vi "Unibot cRIO.vi"() -> ()   [LabVIEW 2012]
uses:
  Unibot - State Machine Controller.vi
  <vilib>/Simulation/Implementation/XNodeFramework/SimXNode/SimX.xnode
  Unibot - Nonlinear Model.vi
  <vilib>/Simulation/Utility/Implementation/SIM Halt.vi
  <vilib>/Simulation/SignalDisplay/Implementation/NILVSim Time Waveform.llb/SIM Time Waveform (scalar).vi
  <vilib>/Simulation/Implementation/Shared/SIMSCR Execution Mode.ctl
  <vilib>/Simulation/Scripting/Companion Diagram/SimConfigNode/_simSolvers.ctl
  <vilib>/Simulation/Scripting/Companion Diagram/SimConfigNode/SimParams.ctl
  <vilib>/Simulation/Scripting/Companion Diagram/SimConfigNode/SimDog.xnode
panel:
  in  "Tab Control":T1(tab)
  in  "Start Open Loop":bool
  out "torque 2":waveform(dbl)(graph)={"t0"=timestamp(0 s since 1904-01-01), "dt"=1.0, "Y"=[0.0]}
  out "teta2 2":waveform(dbl)(graph)={"t0"=timestamp(0 s since 1904-01-01), "dt"=1.0, "Y"=[0.0]}
  out "teta1 2":waveform(dbl)(graph)={"t0"=timestamp(0 s since 1904-01-01), "dt"=1.0, "Y"=[0.0]}
  in  "Initial Theta1 (Elbow)":dbl(knob) scale=-3.14..3.14
  in  "Initial Theta2 (Arm)":dbl(knob) scale=-3.14..3.14
  in  "Right":bool
  in  "Intensity":dbl(slide)=10.0 scale=0.0..10.0
  in  "Left":bool
  in  "Control Technique":T2(tab)
  in  "Q":dbl[][](array[numeric])=[[10.0, 0.0, 0.0, 0.0], [0.0, 10.0, 0.0, 0.0], [0.0, 0.0, 100.0, 0.0], [0.0, 0.0, 0.0, 1.0]] format="%.2f"
  in  "R":dbl[][](array[numeric])=[[50.0]] format="%.2f"
  in  "Desired Pole Location":cdb[](array[numeric])=[0.8275428216771237+0.0i, 0.9068860314786581+0.0i, 0.9511525717602396+0.0i, 0.9425028249515996+0.0i] format="%.2f"
  out "Optimal Gain \nDown-Up":dbl[](array[numeric])=[13.362365480735772, 19.05380394095224, 1.2104119144158012, 2.4013527998190582] format="%.2f"
  out "Optimal Gain\nDown-Down":dbl[](array[numeric])=[-0.14906178101626644, 0.17686358569380023, 1.1761652926773682, -0.039275718443801] format="%.2f"
  out "Optimal Gain \nUp-Up":dbl[](array[numeric])=[-16.081278889113918, -16.397482495141958, -3.1902773104017657, -2.0364914176335533] format="%.2f"
  in  "Type of Control":bool=TRUE
  out "Linearized Equation for Operating Point":picture
  out "Poles locations":cdb[](array[numeric])=[0.6612119646152013+0.0i, 0.9743397418352502+0.0i, 0.9379855295915182+0.0i, 0.9275584671894643+0.0i] format="%.2f"
  out "Impulse Response":cluster{"time":dbl[], dbl[]}[](graph)
  out "Settling Time 1":dbl=2.363776391897807
  out "Settling Time 2":dbl=2.488531257025747
  out "Bode Magnitude":cluster{"W":dbl[], "Magnitude":dbl[]}[](graph)
  out "Bode Phase":cluster{"W":dbl[], "Magnitude":dbl[]}[](graph)
  out "Pole-Zero Map":cluster{dbl[], dbl[]}[](graph)=[{[-30.459733943866535, -2.5043848732190277, -7.159085784207853, -7.159085784207853], [0.0, 0.0, 0.6196593444828095, -0.6196593444828095]}, {[], []}] caption="Closed Loop System Poles"
  out "Stability":T3(ring)
  out "Zeros":cdb[](array[numeric]) format="%.4f"
  out "Poles":cdb[](array[numeric])=[-30.459733943866535+0.0i, -2.5043848732190277+0.0i, -7.159085784207853+0.6196593444828095i, -7.159085784207853-0.6196593444828095i] format="%.4f"
  out "teta1":waveform(dbl)(graph)={"t0"=timestamp(0 s since 1904-01-01), "dt"=1.0, "Y"=[12.566370614359172]}
  out "teta2":waveform(dbl)(graph)={"t0"=timestamp(0 s since 1904-01-01), "dt"=1.0, "Y"=[0.0]}
  out "torque":waveform(dbl)(graph)={"t0"=timestamp(0 s since 1904-01-01), "dt"=1.0, "Y"=[0.0]}
  in  "Halt?":bool
  in  "Kill?":bool
  out "Switching State":string="Bringing home"
  in  "Setpoint":dbl(knob) step=0.01 scale=-0.1..0.1
  in  "Enable?":bool
  in  "Control":bool=TRUE
  in  "PD Gains":T4={"Kp Up"=16.55, "Kd Up"=5.1567, "Kp Down"=10.2, "Kd Down"=0.974}
  # "Pendubot - two link Pendulum with \"elbow\" control"
  # "Objective:"
  # "Pendubot (Pendulum Robot) consists of a DC motor connected to a link physical rigid link (called here 'elbow\") which is connected to a second rigid link ('arm\") that has no actuation (free spinning link).\nThe control objective is to keep the free link in the vertical position while you can choose to balance the controller link (called here elbow) in the extended position (both links are up) or in the contracted position (elbow pointing down and free link up). In those operating points, a State Feedback Control is used to keep in Up-Up or Down-Up position. You can tune those controllers in the Design Tab. The controller also can switch between Down-Down position to any other using state machine to apply another control laws to get to the desired location. The technique used for this operation is called partial feedback linearization and PD controllers were used to implement this system. This example also uses a state-machine to switch between states. To avoid chaotic fall of the pendulum if it can't reach the position, another controller is used to drive the elbow to the stationary position (elbow and free link pointing down)."
  # "Variables:\nTorque (Tau): Voltage applied controller\nTheta1: Encoder Position of the controlled link*\nTheta2: Encoder Position of the free link*\n\n*Enconders have zero reference point down"
  # "Up-Up Position"
  # "Down-Down Position"
  # "Down-Up Position"
  # "In this position, the\nelbow is pointing down and free link is controlled in the up position."
  # "In this position, the elbow and free link are pointing down. This is also a stable position and simulation starts from this point."
  # "In this position, the\nelbow and free link is controlled in the up position, similar to an inverted pendulum."
  # "Disturbance"
  # "Description:"
  # "The allow the system of such complex machine, we need to develop control techniques based on different states. We have a total of 7 controllers that are controlled by a state-macine that switches whenever the condition is stabilished. The \"down-down\"position is considered to be initial state. Whenever the system doesn't meet specific command, the state machine will bring the system to the down-down position. This controller is designed using a Linear Quadratic Regulator with the model linearized at the down-down position. \n\nTo transition between the Down-Down position to Down-Up and Up-Up position, it is used a nonlinear control technique called \"Feedback Linearization\". The implementation of the controller is using a Proportional-Derivative (PD) controller, which is tuned by 'experimentation' in this case.\n\nThe same LQR technique is applied to obtain the controller around the Up-Up and the Down-Up position.  The gain are designed in the 'Control Design' tab and your objective is to choose the gain that makes the controller stable and resistent to disturbance."
  # "State Feedback Controller\nwith state machine"
  # "Initialize"
  # "Swing Up?"
  # "Swing Down?"
  # "Down-Down\nPosition"
  # "Feedback\nlinearization\nPD controller"
  # "Feedback\nlinearization\nPD controller"
  # "Out of\n bounds?"
  # "Out of\n bounds?"
  # "State\nFeedback\nDown-Down"
  # "In bounds?"
  # "In bounds?"
  # "State\nFeedback\nDown-Up"
  # "State\nFeedback\nUp-Up"
  # "Home?"
  # "Home?"
  # "Encoder\nMeasurements\n(Theta1 and Theta 2)"
  # "DC Motor"
  # "State Feedback Controller\nwith state machine"
  # "Swing Up?"
  # "Swing Down?"
  # "Initialize"
  # "Home?"
  # "Home?"
  # "Control Technique"
  # "Desired\nOperating\nPoint"
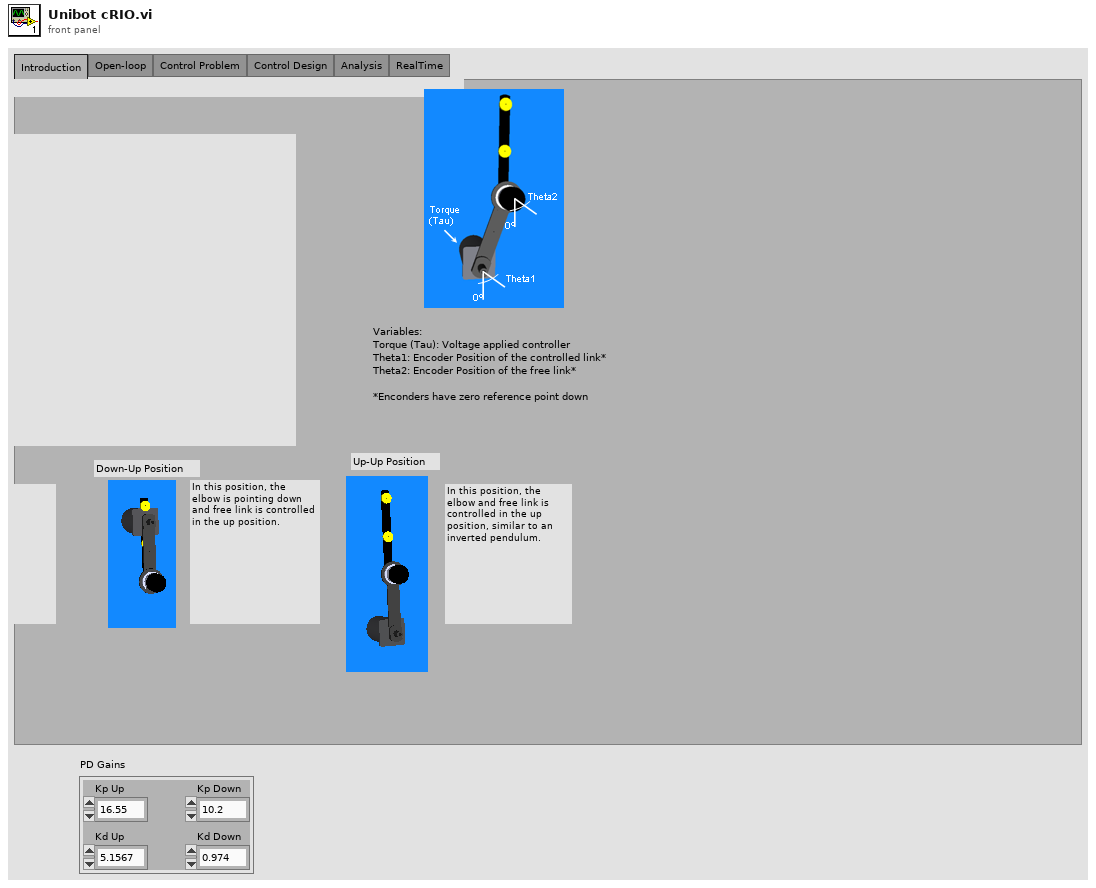
[diagram p1: front panel]
types:
  T1 = enum32{"Introduction", "Open-loop", "Control Problem", "Control Design", "Analysis", "RealTime"}
  T2 = enum32{"Linear Quadratic Regulator", "Pole Placement"}
  T3 = enum16{"stable", "marginally stable", "unstable", "undetermined"}
  T4 = cluster{"Kp Up":dbl, "Kd Up":dbl, "Kp Down":dbl, "Kd Down":dbl}
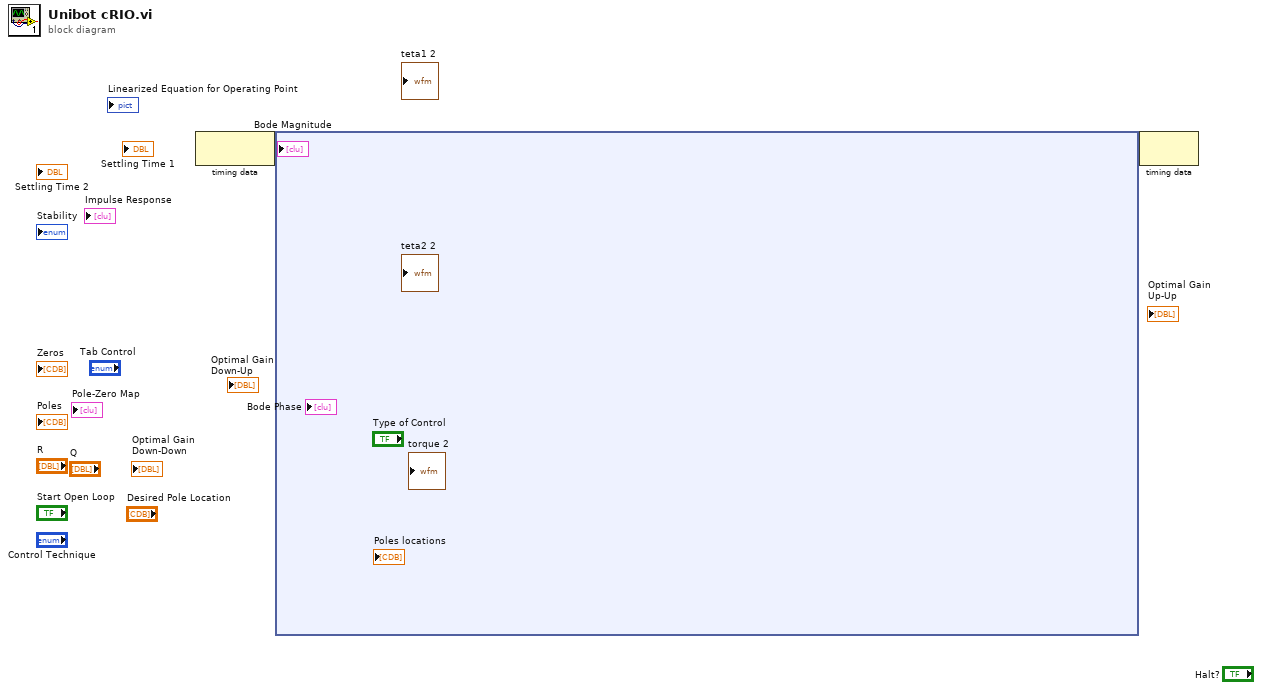
[diagram p0: block diagram]
diagram:
  n1 = node-c288() -> (w2:variant)  [unwired: 1 out]
  n2 = node-c254 ("Simulation Loop 2")(w2) -> (w1:variant)
  n3 = node-c288(w1) -> ()  [unwired: 1 out]
